vi "NIIE_Icon Editor Init Refs.vi"(8 "error in (no error)":errorcluster, 10 "Ref Cluster":T1) -> (0 "error out":errorcluster)   [LabVIEW 2021]
uses:
  Controls/References Cluster.ctl
  MB CORE/TypeDefs/Cluster_Layer Data.ctl
panel:
  in  "Localized tag":string="Import Icon from Owning Library"
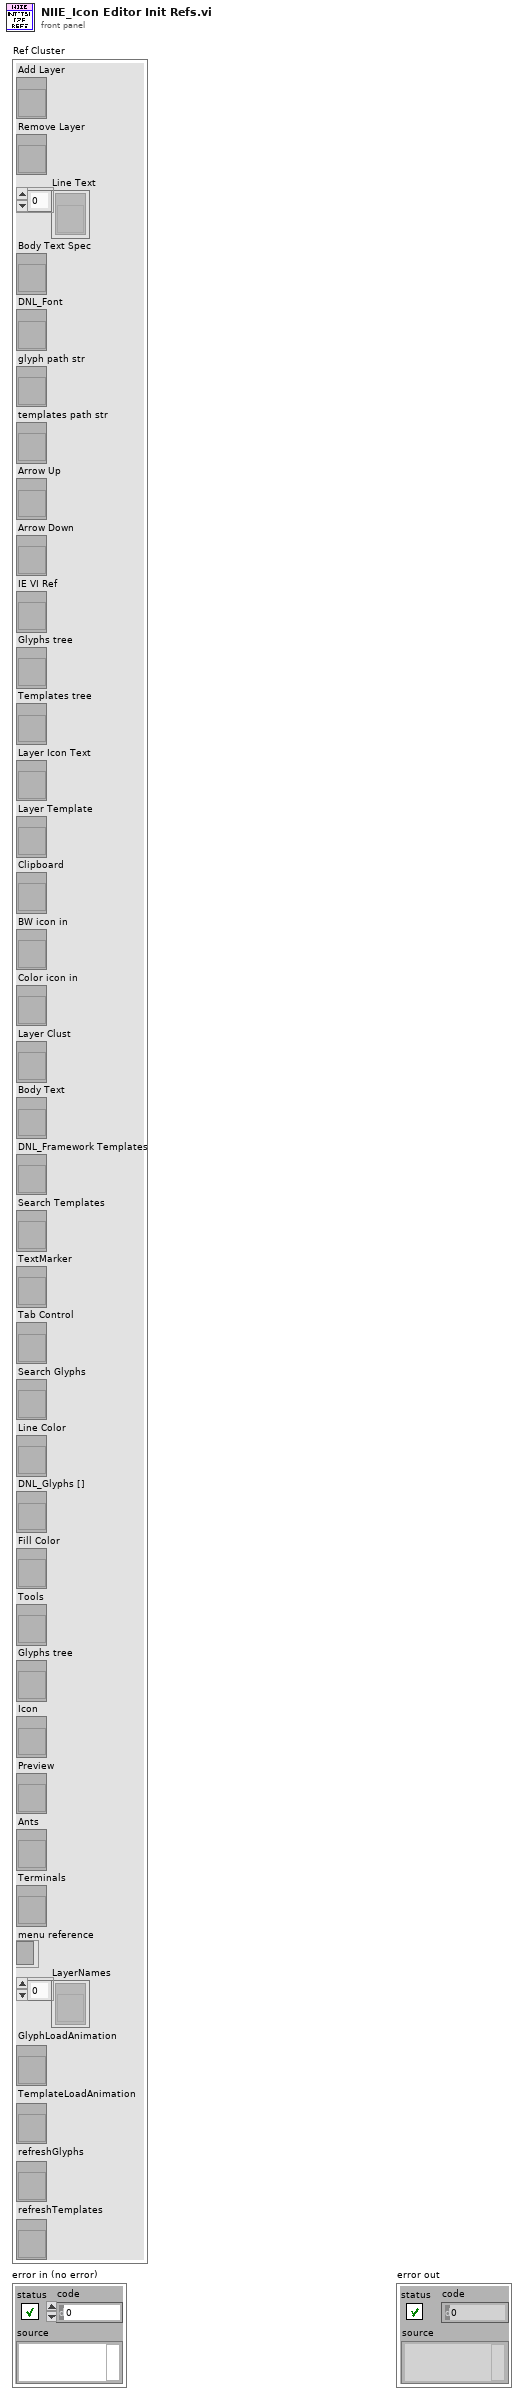
[diagram p1: front panel]
types:
  T1 = typedef "References Cluster.ctl" = cluster{"Add Layer":refnum<vi>, "Remove Layer":refnum<vi>, "Line Text":refnum<vi>[], "Body Text Spec":refnum<vi>, "DNL_Font":refnum<vi>, "glyph path str":refnum<vi>, "templates path str":refnum<vi>, "Arrow Up":refnum<vi>, "Arrow Down":refnum<vi>, "IE VI Ref":refnum<vi>, "Glyphs tree":refnum<vi>, "Templates tree":refnum<vi>, "Layer Icon Text":refnum<vi>, "Layer Template":refnum<vi>, "Clipboard":refnum<vi>, "BW icon in":refnum<vi>, "Color icon in":refnum<vi>, "Layer Clust":refnum<vi>, "Body Text":refnum<vi>, "DNL_Framework Templates":refnum<vi>, "Search Templates":refnum<vi>, "TextMarker":refnum<vi>, "Tab Control":refnum<vi>, "Search Glyphs":refnum<vi>, "Line Color":refnum<vi>, "DNL_Glyphs []":refnum<vi>, "Fill Color":refnum<vi>, "Tools":refnum<vi>, "Glyphs tree":refnum<vi>, "Icon":refnum<vi>, "Preview":refnum<vi>, "Ants":refnum<vi>, "Terminals":refnum<vi>, "menu reference":refnum<k9>, "LayerNames":refnum<vi>[], "GlyphLoadAnimation":refnum<vi>, "TemplateLoadAnimation":refnum<vi>, "refreshGlyphs":refnum<vi>, "refreshTemplates":refnum<vi>}
  T2 = typedef "Cluster_Layer Data.ctl" = cluster{"LayerIcon":picture, "LayerName":string, "Opacity":u8, "Visibility?":bool}
  T3 = typedef "Cluster_INI Data.ctl" = cluster{"Show Layer Tab?":bool, "Show Terminals?":bool, "Text":cluster{"Font":T4, "Alignment":T5, "Size":T6}, "3rd party Templates":cluster{"Store 3rd party Templates?":bool, "Folder Name":string}, "Merge user layers on commit":bool, "Body Text":T7, "Fill Color":T8, "Edge Color":T8, "Tab":u16, "Tool":T9, "Disable Layers?":bool}
  T4 = typedef "Font.ctl" = string
  T5 = typedef "Alignment.ctl" = u16
  T6 = typedef "Num_Font Size.ctl" = u8
  T7 = typedef "Cluster_BodyText.ctl" = cluster{"Line 1 text":string, "Line 2 text":string, "Line 3 text":string, "Line 4 text":string, "Line 1 color":u32, "Line 2 color":u32, "Line 3 color":u32, "Line 4 color":u32, "Body Text Spec":cluster{"Font":T4, "Alignment":T5, "Size":u8}, "Center text vertically":bool, "Capitalize Text":bool}
  T8 = typedef "IEColor.ctl" = u32
  T9 = typedef "Cluster_Button Draw Tools.ctl" = enum32{"Pencil", "Line", "Dropper", "Fill", "Rectangle", "Filled Rectangle", "Ellipse", "Filled Ellipse", "Eraser", "Text", "Select", "Move"}
  T10 = typedef "Who Invoked Icon Editor.ctl" = cluster{"Icon Editor Invoker Type":T11, "App Refnum of Invoker":refnum<vi>, "Qualified Name of Invoker":string, "Path to Invoker":path}
  T11 = typedef "Icon Editor Invoker Type.ctl" = enum32{"Unknown Icon Source", "VI Icon", "Library Icon (any library type)", "Palette icon", "Icon from App Method"}
  T12 = typedef "LabVIEW Icon Stored Information.ctl" = cluster{"Text Visible?":bool, "Text Opacity":u8, "Templ Visible?":bool, "Templ Opacity":u8, "Relative Path from 1 to 2":path, "Image":picture, "All User Layers":refnum<class "Layer.lvclass">[], "Body Text":T7}
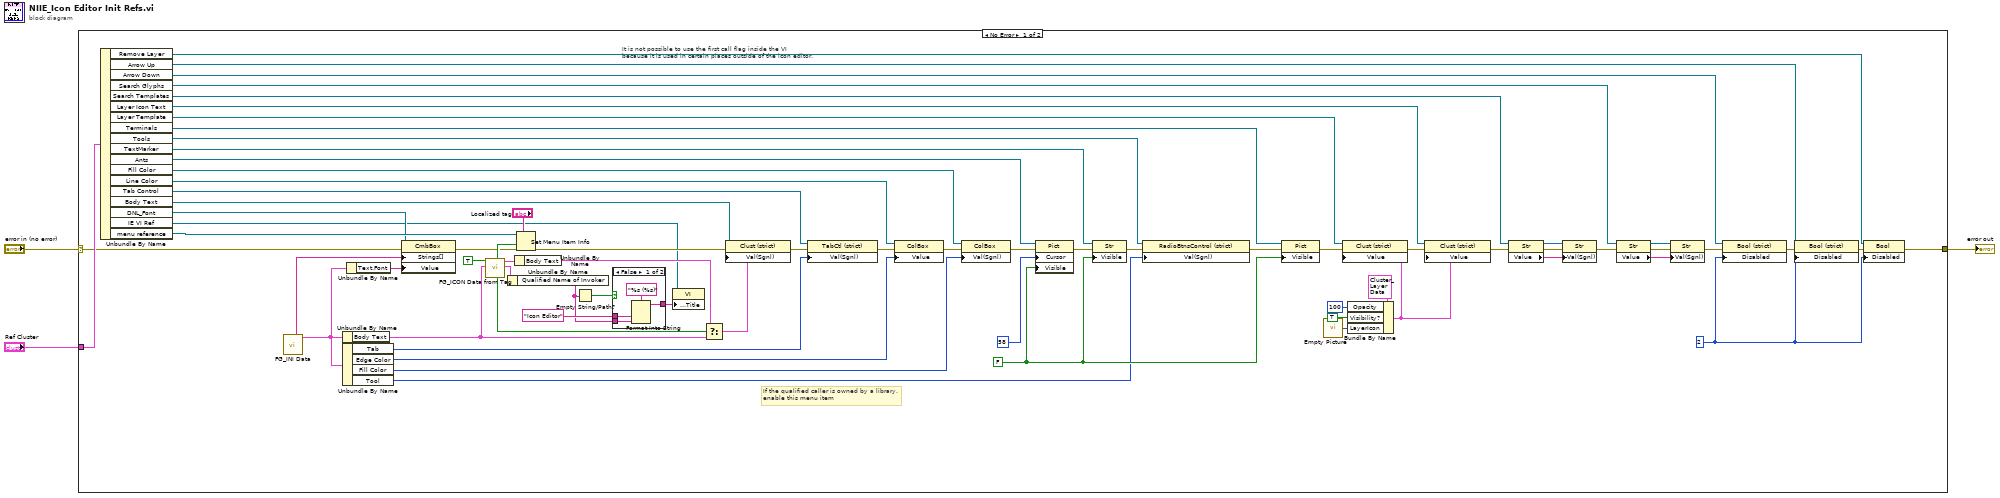
[diagram p0: block diagram]
diagram:
  n1 = case shown="No Error" "error in (no error)" {
    selector: "error in (no error)" -> [w13 w80]
    tunnel: [w23 w80] -> w2
    tunnel: "Ref Cluster" -> [w48 _]
    frame No Error {
      w22 = u8 2 ("Disabled")
      w57 = FALSE ("Visible")
      # "If the qualified caller is owned by a library,\nenable this menu item"
      # "It is not possible to use the first call flag inside the VI\nbecause it is used in certain places outside of the icon editor."
      n2 = Unbundle By Name(w48) -> ("Remove Layer"=w21:refnum<vi>, "Arrow Up"=w46:refnum<vi>, "Arrow Down"=w47:refnum<vi>, "Search Glyphs"=w37:refnum<vi>, "Search Templates"=w44:refnum<vi>, "Layer Icon Text"=w30:refnum<vi>, "Layer Template"=w49:refnum<vi>, "Terminals"=w59:refnum<vi>, "Tools"=w62:refnum<vi>, "TextMarker"=w63:refnum<vi>, "Ants"=w65:refnum<vi>, "Fill Color"=w73:refnum<vi>, "Line Color"=w74:refnum<vi>, "Tab Control"=w56:refnum<vi>, "Body Text"=w27:refnum<vi>, "DNL_Font"=w14:refnum<vi>, "IE VI Ref"=w6:refnum<vi>, "menu reference"=w18:refnum<k9>)
      n3 = call "FG_INI Data.vi"() -> ("INI Data Out"=w11:T3, "Font List Out"=w15:string[])  [unwired: 9 in, 1 out]
      n4 = Unbundle By Name(w11) -> ("Body Text"=w16:T7)
      n5 = Unbundle By Name(w11) -> ("Tab"=w54:u16, "Edge Color"=w71:T8, "Fill Color"=w70:T8, "Tool"=w53:T9)
      n6 = Unbundle By Name(w11) -> ("Text.Font"=w10:T4)
      n7 = property class="CmbBox"(reference=w14, error in=w13, "Strings[]"=w15, "Value"=w10) -> (error out=w12:errorcluster)  [unwired: 1 out]
      n8 = call "FG_ICON Data from Tag.vi"("Default Body Text"=w16, "Init? (F)"=TRUE) -> ("Invoked Data Out"=w5:T10, "Data Out"=w68:T12, "Valid? Out"=w69:bool, "Valid Library Icon? Out"=w19:bool)  [unwired: 1 in, 5 out]
      n9 = Unbundle By Name(w5) -> ("Qualified Name of Invoker"=w4:string)
      n10 = Unbundle By Name(w68) -> ("Body Text"=w67:T7)
      n11 = Set Menu Item Info(7:"Localized tag", 8:w12, 9:w19, 11:w18) -> (0:w17:errorcluster)  [unwired: 3 in, 1 out]
      n12 = Empty String/Path?(string/path=w4) -> (empty?=w8:bool)
      n13 = case shown="False" w8 {
        tunnel: "Icon Editor" ("Localized string") -> [w78 w79]
        tunnel: w4 -> [w76 _]
        tunnel: [w75 w79] -> w9
        frame False {
          n14 = Format Into String(format string="%s (%s)", w78, w76) -> (resulting string=w75:string)  [unwired: 2 in, 1 out]
        }
        frame True {
        }
      }
      n15 = property class="VI"(reference=w6, "Front Panel.Title"=w9) -> ()  [unwired: 1 in, 2 out]
      n16 = Select(t=w67, s=w69, f=w16) -> (s? t:f=w66:T7)
      n17 = property class="Clust (strict)"(reference=w27, error in=w17, "Val(Sgnl)"=w66) -> (error out=w26:errorcluster)  [unwired: 1 out]
      n18 = property class="TabCtl (strict)"(reference=w56, error in=w26, "Val(Sgnl)"=w54) -> (error out=w55:errorcluster)  [unwired: 1 out]
      n19 = property class="ColBox"(reference=w74, error in=w55, "Value"=w71) -> (error out=w72:errorcluster)  [unwired: 1 out]
      n20 = property class="ColBox"(reference=w73, error in=w72, "Val(Sgnl)"=w70) -> (error out=w25:errorcluster)  [unwired: 1 out]
      n21 = property class="Pict"(reference=w65, error in=w25, "Cursor"=58, "Visible"=w57) -> (error out=w61:errorcluster)  [unwired: 1 out]
      n22 = property class="Str"(reference=w63, error in=w61, "Visible"=w57) -> (error out=w60:errorcluster)  [unwired: 1 out]
      n23 = property class="RadioBtnsControl (strict)"(reference=w62, error in=w60, "Val(Sgnl)"=w53) -> (error out=w58:errorcluster)  [unwired: 1 out]
      n24 = property class="Pict"(reference=w59, error in=w58, "Visible"=w57) -> (error out=w50:errorcluster)  [unwired: 1 out]
      n25 = call "Empty Picture"() -> ("empty picture"=w51:picture)
      n26 = Bundle By Name(cluster=T2 {"LayerIcon"=bytes[0], "LayerName"="", "Opacity"=0, "Visibility?"=FALSE} ("Value (Signaling)"), "Opacity"=u8 100, "Visibility?"=TRUE, "LayerIcon"=w51) -> (w29:T2)
      n27 = property class="Clust (strict)"(reference=w49, error in=w50, "Value"=w29) -> (error out=w31:errorcluster)  [unwired: 1 out]
      n28 = property class="Clust (strict)"(reference=w30, error in=w31, "Value"=w29) -> (error out=w28:errorcluster)  [unwired: 1 out]
      n29 = property class="Str"(reference=w44, error in=w28) -> (reference out=w43:refnum<vi>, error out=w42:errorcluster, "Value"=w41:string)
      n30 = property class="Str"(reference=w43, error in=w42, "Val(Sgnl)"=w41) -> (error out=w36:errorcluster)  [unwired: 1 out]
      n31 = property class="Str"(reference=w37, error in=w36) -> (reference out=w38:refnum<vi>, error out=w39:errorcluster, "Value"=w40:string)
      n32 = property class="Str"(reference=w38, error in=w39, "Val(Sgnl)"=w40) -> (error out=w35:errorcluster)  [unwired: 1 out]
      n33 = property class="Bool (strict)"(reference=w47, error in=w35, "Disabled"=w22) -> (error out=w45:errorcluster)  [unwired: 1 out]
      n34 = property class="Bool (strict)"(reference=w46, error in=w45, "Disabled"=w22) -> (error out=w24:errorcluster)  [unwired: 1 out]
      n35 = property class="Bool"(reference=w21, error in=w24, "Disabled"=w22) -> (error out=w23:errorcluster)  [unwired: 1 out]
    }
    frame Error {
    }
  }
  "error out" <- w2
